vi "Init.vi"(8 "error in (no error)":errorcluster, 11 "ArrayController in":refnum<class "ArrayController.lvclass">) -> (0 "error out":errorcluster, 3 "ArrayController out":refnum<class "ArrayController.lvclass">)   [LabVIEW 2019, in "ArrayController.lvclass"]
uses:
  ArrayController.lvclass
  ArrayController.lvclass/ArrayController.ctl
  <vilib>/DAQmx/create/channels.llb/DAQmx Create Channel (AO-Voltage-Basic).vi
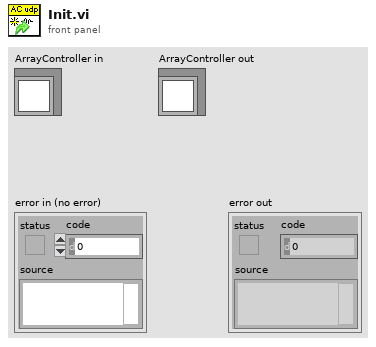
[diagram p1: front panel]
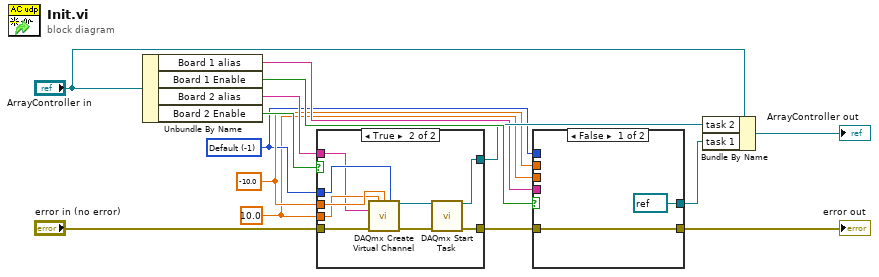
[diagram p0: block diagram]
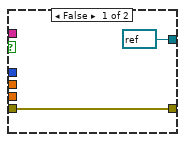
[diagram p2: hidden frame]
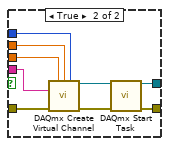
[diagram p3: hidden frame]
diagram:
  w2 = -1 items=["Default"=-1, "RSE"=10083, "Differential"=10106, "Pseudodifferential"=12529] ("output terminal configuration")
  w3 = -10.0 ("minimum value")
  w1 = 10.0 ("maximum value")
  n1 = Unbundle By Name("ArrayController in") -> ("Board 1 alias"=w4:string, "Board 1 Enable"=w10:bool, "Board 2 alias"=w5:string, "Board 2 Enable"=w11:bool)
  n2 = case shown="True" w11 {
    tunnel: [w16 w23] -> w12
    tunnel: [refnum<k21> refnum ("task out") w22] -> w9
    tunnel: "error in (no error)" -> [w16 w21]
    tunnel: w5 -> [_ w17]
    tunnel: w2 -> [_ w20]
    tunnel: w3 -> [_ w19]
    tunnel: w1 -> [_ w18]
    frame False {
    }
    frame True {
      n3 = call-poly <vilib>:"DAQmx Create Virtual Channel.vi"("maximum value"=w18, "minimum value"=w19, "output terminal configuration"=w20, "physical channels"=w17, "error in"=w21) -> ("task out"=w24:refnum<k21>, "error out"=w25:errorcluster)  [unwired: 9 in]
      n4 = call <vilib>:"DAQmx Start Task.vi"("task/channels in"=w24, "error in"=w25) -> ("task out"=w22:refnum<k21>, "error out"=w23:errorcluster)  [unwired: 12 in]
    }
  }
  n5 = case shown="False" w10 {
    tunnel: [refnum<k21> refnum ("task out") w34] -> w8
    tunnel: w12 -> [w27 w33]
    tunnel: [w27 w32] -> w7
    tunnel: w4 -> [_ w31]
    tunnel: w3 -> [_ w30]
    tunnel: w2 -> [_ w29]
    tunnel: w1 -> [_ w28]
    frame False {
    }
    frame True {
      n6 = call-poly <vilib>:"DAQmx Create Virtual Channel.vi"("maximum value"=w28, "minimum value"=w30, "output terminal configuration"=w29, "physical channels"=w31, "error in"=w33) -> ("task out"=w36:refnum<k21>, "error out"=w35:errorcluster)  [unwired: 9 in]
      n7 = call <vilib>:"DAQmx Start Task.vi"("task/channels in"=w36, "error in"=w35) -> ("task out"=w34:refnum<k21>, "error out"=w32:errorcluster)  [unwired: 12 in]
    }
  }
  "error out" <- w7
  n8 = Bundle By Name(cluster="ArrayController in", "task 2"=w9, "task 1"=w8) -> (→"ArrayController out":refnum<class "ArrayController.lvclass">)
